vi "rad_Compare Checksums.vi"(10 "Checksums 2":cluster{path, string}[](array[cluster]), 11 "Checksums 1":cluster{path, string}[](array[cluster])) -> (0 "Files In 2 Only":path[](array[path]), 1 "Files In 1 Only":path[](array[path]), 2 "Modified Files":path[](array[path]), 3 "Identical?":bool)   [LabVIEW 2020]
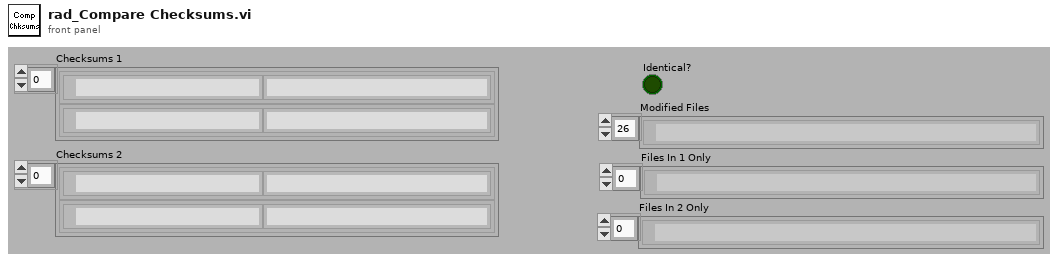
[diagram p1: front panel]
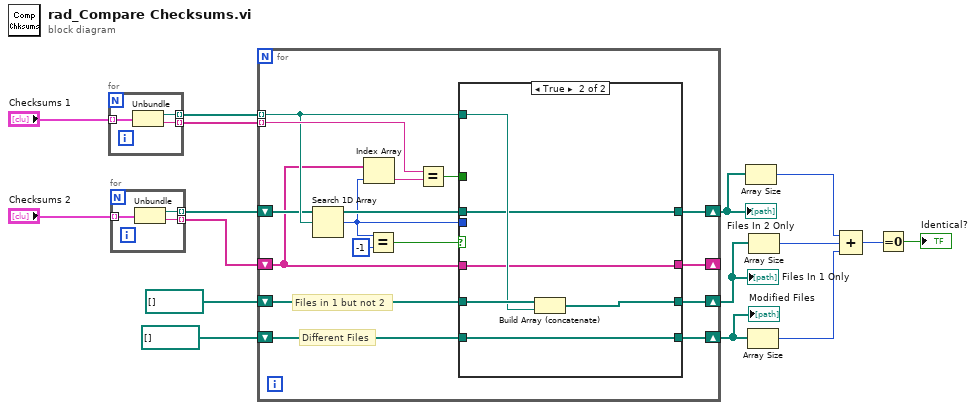
[diagram p0: block diagram]
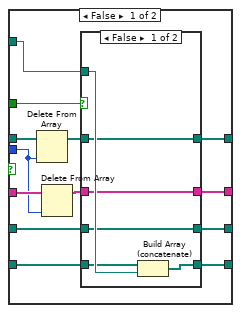
[diagram p2: hidden frame]
diagram:
  n1 = for {
    tunnel: "Checksums 1" -> [w19] mode=indexing
    tunnel: [w18] -> w13 mode=indexing
    tunnel: [w17] -> w14 mode=indexing
    n2 = Unbundle(w19) -> (w18:path, w17:string)
  }
  n3 = for {
    tunnel: [w20] -> _ mode=indexing
    tunnel: [w22] -> w12 mode=indexing
    tunnel: [w21] -> w11 mode=indexing
    tunnel: "Checksums 2" -> [w20] mode=indexing
    n4 = Unbundle(w20) -> (w22:path, w21:string)
  }
  n5 = for {
    tunnel: w14 -> [w37] mode=indexing
    tunnel: w13 -> [w33] mode=indexing
    shift-right: [w31] -> w7
    shift-left: path[] [] -> [w32]
    shift-right: [w25] -> w6
    shift-left: path[] [] -> [w26]
    shift-right: [w29] -> w8
    shift-left: w12 -> [w28]
    shift-right: [w23] -> _
    shift-left: w11 -> [w24]
    # "Files in 1 but not 2"
    # "Different Files"
    n6 = Search 1D Array(1D array=w28, element=w33) -> (index of element=w27:i32)  [unwired: 1 out]
    n7 = Index Array(array=w24, index=w27) -> (element=w36:string)
    n8 = Equal?(x=w27, y=-1) -> (x = y?=w34:bool)
    n9 = Equal?(x=w37, y=w36) -> (x = y?=w30:bool)
    n10 = case shown="True" w34 {
      tunnel: w33 -> [w46 w65]
      tunnel: w32 -> [w43 w66]
      tunnel: [w44 w64] -> w31
      tunnel: w30 -> [w50 _]
      tunnel: [w49 w63] -> w29
      tunnel: w28 -> [w48 w63]
      tunnel: w27 -> [w40 _]
      tunnel: w26 -> [w45 w62]
      tunnel: [w42 w62] -> w25
      tunnel: w24 -> [w41 w61]
      tunnel: [w39 w61] -> w23
      frame False {
        n11 = Delete From Array(array=w48, index=w40) -> (array with subset deleted=w47:path[])  [unwired: 1 in, 1 out]
        n12 = Delete From Array(array=w41, index=w40) -> (array with subset deleted=w38:string[])  [unwired: 1 in, 1 out]
        n13 = case shown="False" w50 {
          tunnel: [w52 w60] -> w49
          tunnel: w47 -> [w52 w60]
          tunnel: w46 -> [w56 _]
          tunnel: w45 -> [w55 w58]
          tunnel: [w54 w59] -> w44
          tunnel: w43 -> [w54 w59]
          tunnel: [w53 w58] -> w42
          tunnel: [w51 w57] -> w39
          tunnel: w38 -> [w51 w57]
          frame False {
            n14 = Build Array (concatenate)(w55, w56) -> (w53:path[])
          }
          frame True {
          }
        }
      }
      frame True {
        n15 = Build Array (concatenate)(w66, w65) -> (w64:path[])
      }
    }
  }
  "Files In 2 Only" <- w8
  "Files In 1 Only" <- w7
  "Modified Files" <- w6
  n16 = Array Size(array=w8) -> (size(s)=w5:i32)
  n17 = Array Size(array=w6) -> (size(s)=w3:i32)
  n18 = Array Size(array=w7) -> (size(s)=w4:i32)
  n19 = Compound Arithmetic op=ADD(w5, w4, w3) -> (w2:i32)
  n20 = Equal To 0?(x=w2) -> (x = 0?=→"Identical?":bool)
